vi "SystemVolume.Set.vi"(6 "Mode":i32(ring)=2 items=["Render", "Capture", "All"], 8 "error in (no error)":errorcluster, 10 "Volumes":i32[](array[numeric]), 11 "FriendlyName (\"\": All)":string) -> (0 "error out":errorcluster, 2 "FriendlyNames":string[](array[string]))   [LabVIEW 2014]
uses:
  C:/Program Files (x86)/National Instruments/LabVIEW 2014/user.lib/dge-library/LabVIEW/System/SystemVolume/NAudio.dll
  NAudio.dll
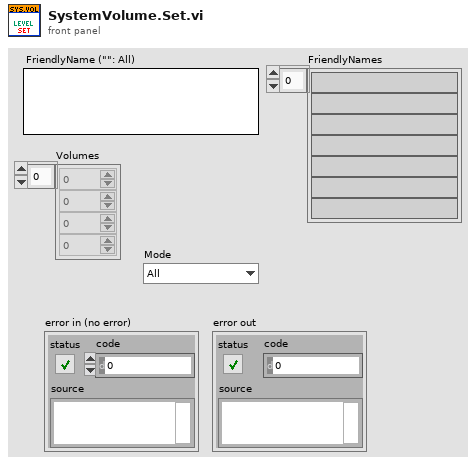
[diagram p1: front panel]
types:
  T1 = cluster{"AudioClient":refnum<k24>, "AudioEndpointVolume":refnum<k24>, "AudioMeterInformation":refnum<k24>, "AudioSessionManager":refnum<k24>, "DataFlow":i32, "DeviceFriendlyName":string, "FriendlyName":string, "IconPath":string, "ID":string}[]
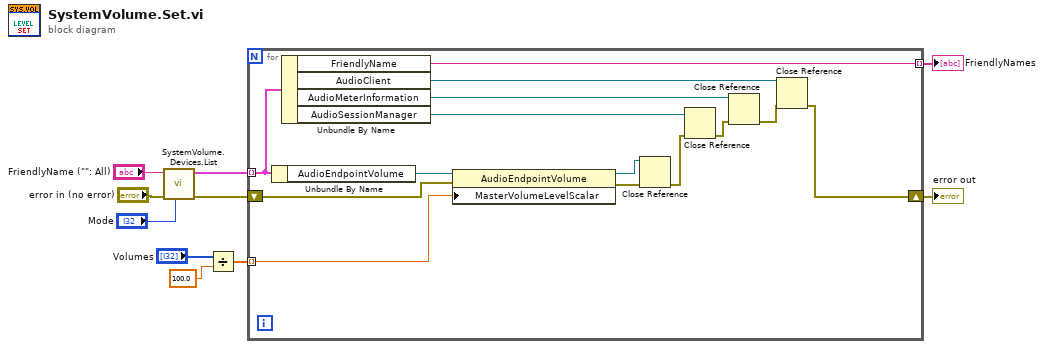
[diagram p0: block diagram]
diagram:
  n1 = call <userlib>:"SystemVolume.Devices.List.vi"("dataFlow"="Mode", "error in (no error)"="error in (no error)", "FriendlyName (\"\": All)"="FriendlyName (\"\": All)") -> ("error out"=w9:errorcluster, "Info"=w10:T1)  [unwired: 7 in]
  n2 = Divide(x="Volumes", y=sgl 100.0) -> (x/y=w3:sgl[])
  n3 = for {
    tunnel: w10 -> [w21] mode=indexing
    shift-right: [w14] -> w8
    shift-left: w9 -> [w13]
    tunnel: [w12] -> w6 mode=indexing
    tunnel: w3 -> [w11] mode=indexing
    n4 = Unbundle By Name(w21) -> ("AudioEndpointVolume"=w22:refnum<k24>)
    n5 = Unbundle By Name(w21) -> ("FriendlyName"=w12:string, "AudioClient"=w20:refnum<k24>, "AudioMeterInformation"=w19:refnum<k24>, "AudioSessionManager"=w17:refnum<k24>)
    n6 = property class="AudioEndpointVolume"(reference=w22, error in=w13, "MasterVolumeLevelScalar"=w11) -> (reference out=w24:refnum<k24>, error out=w23:errorcluster)
    n7 = Close Reference(reference=w24, error in (no error)=w23) -> (error out=w15:errorcluster)
    n8 = Close Reference(reference=w17, error in (no error)=w15) -> (error out=w16:errorcluster)
    n9 = Close Reference(reference=w19, error in (no error)=w16) -> (error out=w18:errorcluster)
    n10 = Close Reference(reference=w20, error in (no error)=w18) -> (error out=w14:errorcluster)
  }
  "error out" <- w8
  "FriendlyNames" <- w6
